vi "Select Positions from ENUM.vi"(7 "PoseList":T1={"MotionMaster Ver"=0, "Pose List"=[{"Pose"=enum."None-Unknown", "Target"={"Sholder"=0, "Extend"=0, "Wrist"=0}}, {"Pose"=enum."Intake", "Target"={"Sholder"=326, "Extend"=-6481, "Wrist"=723}}, {"Pose"=enum."Score High", "Target"={"Sholder"=970, "Extend"=-11200, "Wrist"=810}}, {"Pose"=enum."Score Mid", "Target"={"Sholder"=910, "Extend"=-3500, "Wrist"=1417}}, {"Pose"=enum."Safe Position", "Target"={"Sholder"=500, "Extend"=-500, "Wrist"=10}}, {"Pose"=enum."Home Pos", "Target"={"Sholder"=154, "Extend"=-500, "Wrist"=10}}]}, 11 "Pose":T3) -> (3 "Selectet  Position Out":T4={"Sholder"=154, "Extend"=-50, "Wrist"=10})   [LabVIEW 2020]
uses:
  ENUM_Pose List.ctl
  Shared Code/TypeDefs/Cluster_Pose Positions.ctl
  Shared Code/TypeDefs/Cluster_MotionMaster_Config Data.ctl
  Shared Code/TypeDefs/Cluster_Pose Name and  Data.ctl
  4ff530dc-51a0-4cd1-8eb0-b86096a80c95.vi
  MotionMaster_SubCMD.lvlib
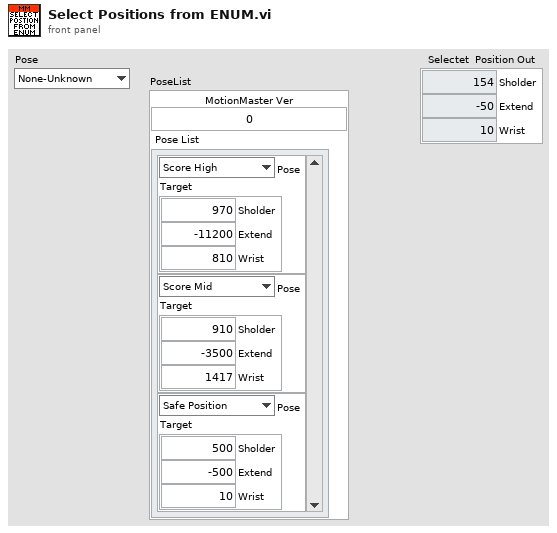
[diagram p1: front panel]
types:
  T1 = typedef "Cluster_MotionMaster_Config Data.ctl" = cluster{"MotionMaster Ver":u64, "Pose List":T2[]}
  T2 = typedef "Cluster_Pose Name and  Data.ctl" = cluster{"Pose":T3, "Target":T4}
  T3 = typedef "MotionMaster_SubCMD.lvlib/ENUM_Pose List.ctl" = enum16{"None-Unknown", "Intake", "Score High", "Score Mid", "Safe Position", "Home Pos"}
  T4 = typedef "Cluster_Pose Positions.ctl" = cluster{"Sholder":i32, "Extend":i32, "Wrist":i32}
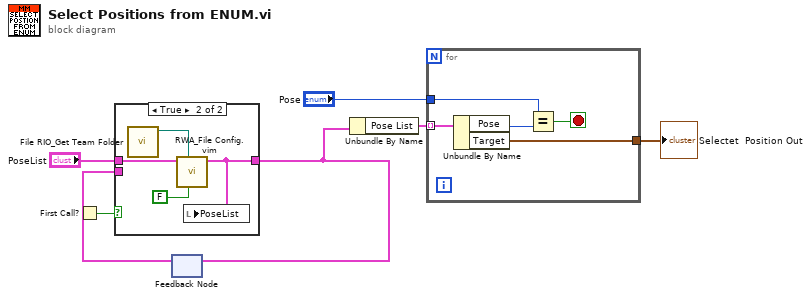
[diagram p0: block diagram]
diagram:
  n1 = First Call?() -> (First Call?: T/F=w2:bool)
  n2 = feedback #1() -> (w1:T1)  [unwired: 1 in]
  n3 = case shown="True" w2 {
    tunnel: "PoseList" -> [_ w11]
    tunnel: [w8 w9] -> w3
    tunnel: w1 -> [w8 _]
    frame False {
    }
    frame True {
      n4 = call "File RIO_Get Team Folder.vi"() -> ("Team Files Folder"=w10:path)  [unwired: 10 in, 1 out]
      n5 = call "RWA_File Config.vim"("Read(f) Write(t)"=FALSE, "Target Folder Folder"=w10, "Any Config"=w11) -> ("Any Config Out"=w9:T1)  [unwired: 4 in, 4 out]
      n6 = local write "PoseList"(w9) -> ()
    }
  }
  n7 = feedback-in #1(w3) -> ()
  n8 = Unbundle By Name(w3) -> ("Pose List"=w6:T2[])
  n9 = for {
    tunnel: "Pose" -> [w15]
    tunnel: w6 -> [w17] mode=indexing
    tunnel: [w13] -> w5
    stop <- w14 stop-if-true
    n10 = Unbundle By Name(w17) -> ("Pose"=w16:T3, "Target"=w13:T4)
    n11 = Equal?(x=w15, y=w16) -> (x = y?=w14:bool)
  }
  "Selectet  Position Out" <- w5
